vi "ConvertSetNames.vi"(11 "Set Names":string) -> (3 "Set Names":string[](array[string]))   [LabVIEW 2022 SP3]
uses:
  <vilib>/Utility/error.llb/Trim Whitespace One-Sided.vi
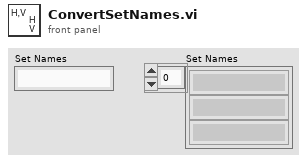
[diagram p1: front panel]
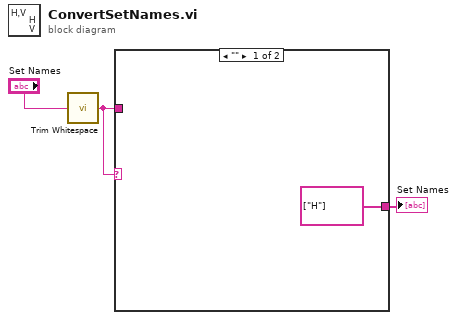
[diagram p0: block diagram]
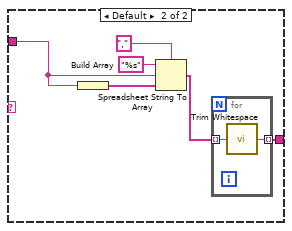
[diagram p2: hidden frame]
diagram:
  n1 = call <vilib>:"Trim Whitespace.vi"("string"="Set Names") -> ("trimmed string"=w1:string)  [unwired: 1 in]
  n2 = case shown="\"\"" w1 {
    tunnel: [string[] ["H"] w6] -> w3
    tunnel: w1 -> [_ w5]
    frame "" {
    }
    frame Default {
      n3 = Build Array(w5) -> (w10:string[])
      n4 = Spreadsheet String To Array(delimiter (Tab)=",", format string="%s", spreadsheet string=w5, array type (2D Dbl)=w10) -> (array=w7:string[])
      n5 = for {
        tunnel: w7 -> [w12] mode=indexing
        tunnel: [w11] -> w6 mode=indexing
        n6 = call <vilib>:"Trim Whitespace.vi"("string"=w12) -> ("trimmed string"=w11:string)  [unwired: 1 in]
      }
    }
  }
  "Set Names" <- w3
